vi "Write Source.vi"(8 "Error In":errorcluster, 10 "Source":string, 11 "Token In":refnum<class "Abstract.lvclass">) -> (0 "Error Out":errorcluster, 3 "Token Out":refnum<class "Abstract.lvclass">)   [LabVIEW 2018]
uses:
  Abstract.lvclass
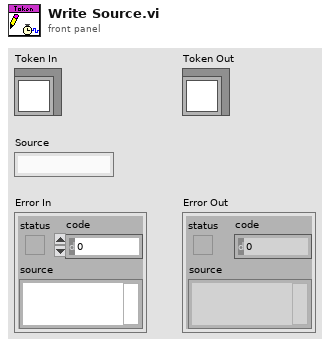
[diagram p1: front panel]
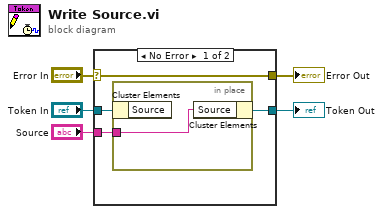
[diagram p0: block diagram]
diagram:
  n1 = case shown="No Error" "Error In" {
    selector: "Error In" -> [w9 w11]
    tunnel: [w9 w11] -> w4
    tunnel: [w6 w12] -> w2
    tunnel: "Token In" -> [w8 w12]
    tunnel: "Source" -> [w7 _]
    frame No Error {
      n2 = in-place {
        in-place-border: w7 -> [w10]
        n3 = in-place-cluster #1(w8) -> ()  [unwired: 1 out]
        n4 = in-place-cluster #1("Source"=w10) -> (w6:refnum<class "Abstract.lvclass">)
      }
    }
    frame Error {
    }
  }
  "Error Out" <- w4
  "Token Out" <- w2
